vi "Bus Interface.vi"(0 "niUSRP Rx Core v1 FPGA":refnum<class "niUSRP Sync v1 FPGA.lvclass">, 1 "abort":bool, 5 "instruction":T2, 9 "input valid":bool) -> (6 "response":T1, 10 "done":bool, 14 "ready for input":bool)   [LabVIEW 2025, in "niUSRP Sync v1 FPGA.lvclass"]
uses:
  niUSRP Sync v1 FPGA.lvclass
  <instrlib>/_niInstr/Instruction Framework/v1/FPGA/Interfaces/Address Space/Address Space Instruction.ctl
  <instrlib>/_niInstr/Instruction Framework/v1/FPGA/Typedefs/Response.ctl
  niUSRP Sync v1 FPGA.lvclass/niUSRP Sync v1 FPGA.ctl
  <vilib>/rvi/DataTransferAndStorage/Container/Common/niFpgaContainerExecOnDevCompGetState.vi
  <vilib>/rvi/Emulation/niFpgaEmulationIsFPGAContextNoSignature.vi
  <vilib>/rvi/DataTransferAndStorage/Container/Common/niFpgaContainerGetUniqueNameForEmu.vi
  <vilib>/rvi/Memory/Memory_Emulation/niFpgaMemoryEmulationCacheClearOnFirstRun.vi
  <vilib>/rvi/Memory/Memory_Emulation/nirvimemoryEmulationManagerCache_MakeExclusive.vi
  <vilib>/rvi/Memory/Memory_Emulation/niFpgaMemoryEmulationValidateCache.vi
  <vilib>/rvi/Memory/Memory_Emulation/nirvimemoryEmulationManagerCache_InsertValue.vi
  <vilib>/Utility/error.llb/Clear Errors.vi
  <vilib>/rvi/Memory/Memory_Emulation/nirvimemoryEmulationManagerCache_ReleaseExclusive.vi
  <vilib>/rvi/Memory/Memory_Emulation/nirvimemoryEmulationManagerCache_GetValue.vi
  <vilib>/rvi/Memory/Memory_Emulation/nirvimemoryEmulationManagerCache_SetValue.vi
  <vilib>/rvi/Emulation/niFpgaProcessEmulError.vi
  <vilib>/rvi/Emulation/niFpgaSctlEmulationGetInTimedLoop.vi
  <vilib>/rvi/DataTransferAndStorage/Container/XNode/niFpgaContainer.xnode
  <vilib>/rvi/DataTransferAndStorage/Register/Emulation/niFpgaRegisterEmulationRefIn.vi
  <instrlib>/_niInstr/Instruction Framework/v1/FPGA/Typedefs/niInstr Instruction Framework v1 FPGA.lvlib
  <instrlib>/_niInstr/Basic Elements/v1/FPGA/niInstr Basic Elements v1 FPGA.lvlib
  <instrlib>/_niInstr/Instruction Framework/v1/FPGA/Interfaces/Address Space/Address Space.lvclass
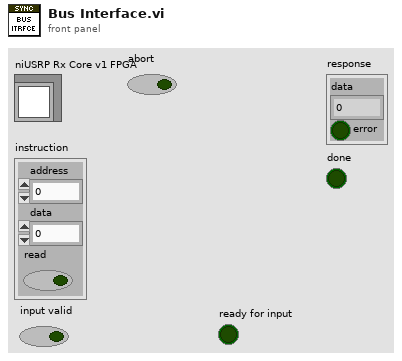
[diagram p1: front panel]
types:
  T1 = typedef "niInstr Instruction Framework v1 FPGA.lvlib/Response.ctl" = cluster{"data":u64, "error":bool}
  T2 = typedef "niInstr Instruction Framework Interfaces v1 FPGA.lvlib/Address Space.lvclass/Address Space Instruction.ctl" = cluster{"address":u32, "data":u64, "read":bool}
  T3 = typedef "niUSRP Sync v1 FPGA.lvclass/Regs.ctl" = cluster{"reset":refnum<k21>, "trigger enable":refnum<k21>, "trigger sync enable":refnum<k21>, "software trigger":refnum<k21>, "trigger select (U8)":refnum<k21>, "trigger out latch 0":refnum<k21>, "trigger out latch 1":refnum<k21>, "trigger time":refnum<k21>, "set trigger time":refnum<k21>, "clear trigger time":refnum<k21>, "time trigger ready":refnum<k21>, "time trigger set in past":refnum<k21>}
  T4 = enum8{"Software", "Digital Edge", "Rx Start Trigger", "Tx Start Trigger", "Immediate", "Future Time Event"}
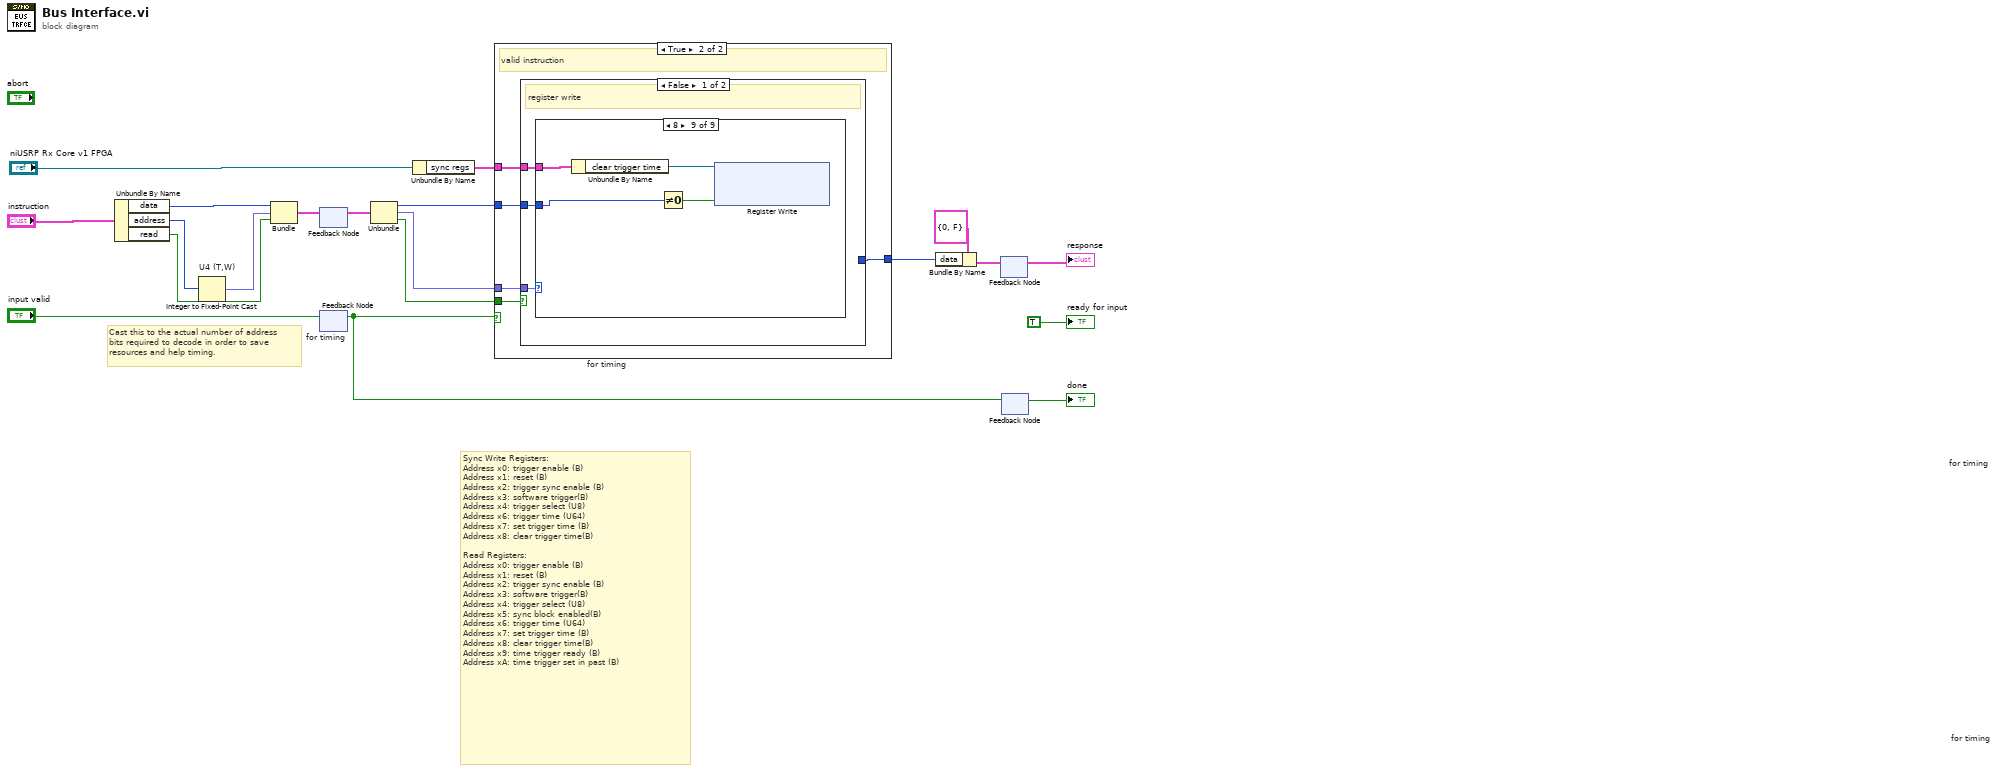
[diagram p0: block diagram]
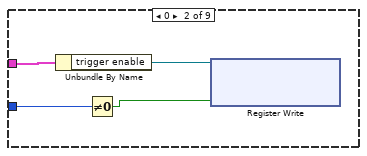
[diagram p4: hidden frame]
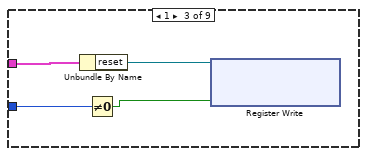
[diagram p5: hidden frame]
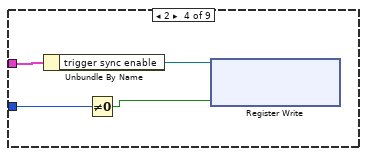
[diagram p6: hidden frame]
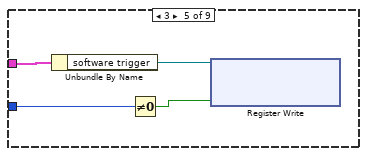
[diagram p7: hidden frame]
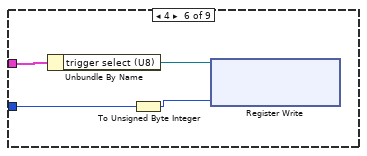
[diagram p8: hidden frame]
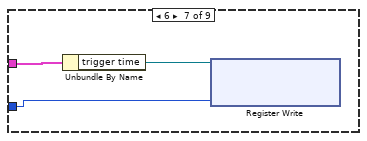
[diagram p9: hidden frame]
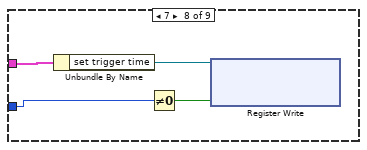
[diagram p10: hidden frame]
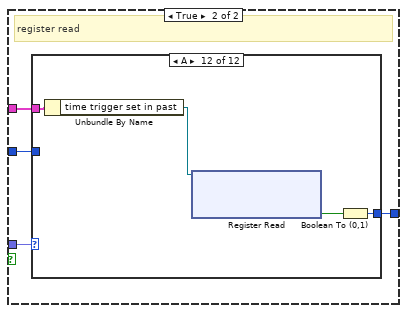
[diagram p11: hidden frame]
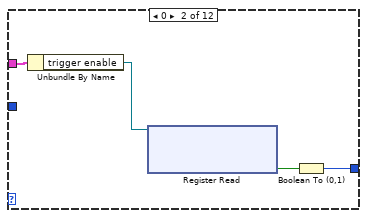
[diagram p13: hidden frame]
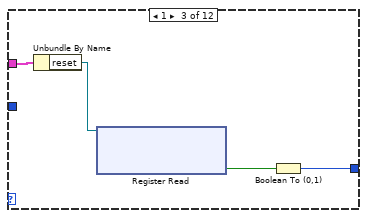
[diagram p14: hidden frame]
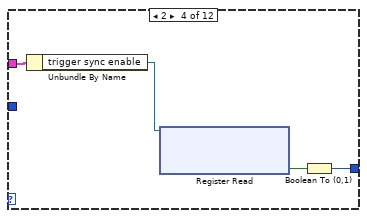
[diagram p15: hidden frame]
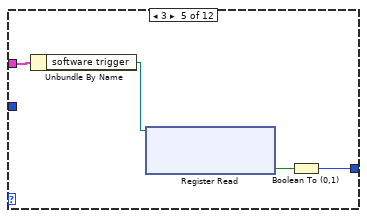
[diagram p16: hidden frame]
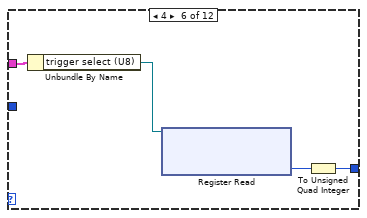
[diagram p17: hidden frame]
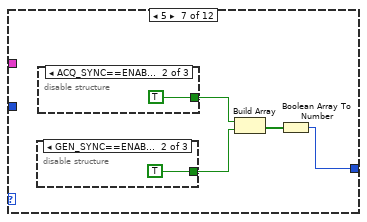
[diagram p18: hidden frame]
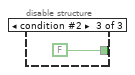
[diagram p20: hidden frame]
diagram:
  # "Sync Write Registers:\nAddress x0: trigger enable (B)\nAddress x1: reset (B)\nAddress x2: trigger sync enable (B)\nAddress x3: software trigger(B)\nAddress x4: trigger select (U8)\nAddress x6: trigger time (U64)\nAddress x7: set trigger time (B)\nAddress x8: clear trigger time(B)\n\nRead Registers:\nAddress x0: trigger enable (B)\nAddress x1: reset (B)\nAddress x2: trigger sync enable (B)\nAddress x3: software trigger(B)\nAddress x4: trigger select (U8)\nAddress x5: sync block enabled(B)\nAddress x6: trigger time (U64)\nAddress x7: set trigger time (B)\nAddress x8: clear trigger time(B)\nAddress x9: time trigger ready (B)\nAddress xA: time trigger set in past (B)"
  # "Cast this to the actual number of address\nbits required to decode in order to save\nresources and help timing."
  n1 = Unbundle By Name("instruction") -> ("data"=w17:u64, "address"=w20:u32, "read"=w15:bool)
  n2 = Integer to Fixed-Point Cast "U4 (T,W)"(integer=w20) -> (fixed-point=w16:fxp<+,4,4>)  [unwired: 1 in]
  n3 = Bundle("data"=w17, w16, "read"=w15) -> (w19:cluster{"data":u64, fxp<+,4,4>, "read":bool})  [unwired: 1 in]
  n4 = feedback #1 "for timing"() -> (w18:cluster{"data":u64, fxp<+,4,4>, "read":bool})  [unwired: 1 in]
  n5 = feedback-in #1(w19) -> ()
  n6 = feedback #2 "for timing"() -> (w1:bool)  [unwired: 1 in]
  n7 = feedback-in #2("input valid") -> ()
  n8 = Unbundle(w18) -> ("data"=w8:u64, w9:fxp<+,4,4>, "read"=w10:bool)
  n9 = Unbundle By Name("niUSRP Rx Core v1 FPGA") -> ("sync regs"=w11:T3)
  n10 = case shown="True" w1 {
    tunnel: w11 -> [_ w25]
    tunnel: w10 -> [_ w24]
    tunnel: w9 -> [_ w23]
    tunnel: w8 -> [_ w22]
    tunnel: [_ w21] -> w7
    frame False {
      # "invalid instruction"
    }
    frame True {
      # "valid instruction"
      n11 = case shown="False" w24 {
        tunnel: w23 -> [w28 w63]
        tunnel: [_ w60] -> w21
        tunnel: w22 -> [w27 w62]
        tunnel: w25 -> [w26 w61]
        frame False {
          # "register write"
          n12 = case shown="8" w28 {
            tunnel: w27 -> [_ w30 w34 w38 w42 w46 w49 w53 w57]
            tunnel: w26 -> [_ w31 w35 w39 w43 w47 w50 w54 w58]
            frame Default {
              # "non-existent register"
            }
            frame 0 {
              n13 = Unbundle By Name(w31) -> ("trigger enable"=w32:refnum<k21>)
              n14 = Not Equal To 0?(x=w30) -> (x != 0?=w29:bool)
              n15 = xnode ("Register Write")("Data"=w29, "Register In"=w32) -> ()  [unwired: 1 out]
            }
            frame 1 {
              n16 = Unbundle By Name(w35) -> ("reset"=w36:refnum<k21>)
              n17 = Not Equal To 0?(x=w34) -> (x != 0?=w33:bool)
              n18 = xnode ("Register Write")("Data"=w33, "Register In"=w36) -> ()  [unwired: 1 out]
            }
            frame 2 {
              n19 = Unbundle By Name(w39) -> ("trigger sync enable"=w40:refnum<k21>)
              n20 = Not Equal To 0?(x=w38) -> (x != 0?=w37:bool)
              n21 = xnode ("Register Write")("Data"=w37, "Register In"=w40) -> ()  [unwired: 1 out]
            }
            frame 3 {
              n22 = Unbundle By Name(w43) -> ("software trigger"=w44:refnum<k21>)
              n23 = Not Equal To 0?(x=w42) -> (x != 0?=w41:bool)
              n24 = xnode ("Register Write")("Data"=w41, "Register In"=w44) -> ()  [unwired: 1 out]
            }
            frame 4 {
              n25 = Unbundle By Name(w47) -> ("trigger select (U8)"=w48:refnum<k21>)
              n26 = To Unsigned Byte Integer(number=w46) -> (unsigned 8bit integer=w45:u8)
              n27 = xnode ("Register Write")("Data"=w45, "Register In"=w48) -> ()  [unwired: 1 out]
            }
            frame 6 {
              n28 = Unbundle By Name(w50) -> ("trigger time"=w51:refnum<k21>)
              n29 = xnode ("Register Write")("Data"=w49, "Register In"=w51) -> ()  [unwired: 1 out]
            }
            frame 7 {
              n30 = Unbundle By Name(w54) -> ("set trigger time"=w55:refnum<k21>)
              n31 = Not Equal To 0?(x=w53) -> (x != 0?=w52:bool)
              n32 = xnode ("Register Write")("Data"=w52, "Register In"=w55) -> ()  [unwired: 1 out]
            }
            frame 8 {
              n33 = Unbundle By Name(w58) -> ("clear trigger time"=w59:refnum<k21>)
              n34 = Not Equal To 0?(x=w57) -> (x != 0?=w56:bool)
              n35 = xnode ("Register Write")("Data"=w56, "Register In"=w59) -> ()  [unwired: 1 out]
            }
          }
        }
        frame True {
          # "register read"
          n36 = case shown="A" w63 {
            tunnel: w62 -> [_ _ _ _ _ _ _ _ _ _ _ _]
            tunnel: w61 -> [_ w66 w70 w74 w79 w82 _ w96 w100 w104 w108 w112]
            tunnel: [_ w64 w68 w72 w78 w80 w84 w97 w99 w103 w107 w111] -> w60
            frame Default {
              # "non-existent register"
            }
            frame 0 {
              n37 = Unbundle By Name(w66) -> ("trigger enable"=w67:refnum<k21>)
              n38 = xnode ("Register Read")("Register In"=w67) -> ("Data"=w65:bool)  [unwired: 1 out]
              n39 = Boolean To (0,1)(Boolean=w65) -> (0, 1=w64:i16)
            }
            frame 1 {
              n40 = Unbundle By Name(w70) -> ("reset"=w71:refnum<k21>)
              n41 = xnode ("Register Read")("Register In"=w71) -> ("Data"=w69:bool)  [unwired: 1 out]
              n42 = Boolean To (0,1)(Boolean=w69) -> (0, 1=w68:i16)
            }
            frame 2 {
              n43 = Unbundle By Name(w74) -> ("trigger sync enable"=w75:refnum<k21>)
              n44 = xnode ("Register Read")("Register In"=w75) -> ("Data"=w73:bool)  [unwired: 1 out]
              n45 = Boolean To (0,1)(Boolean=w73) -> (0, 1=w72:i16)
            }
            frame 3 {
              n46 = Unbundle By Name(w79) -> ("software trigger"=w77:refnum<k21>)
              n47 = xnode ("Register Read")("Register In"=w77) -> ("Data"=w76:bool)  [unwired: 1 out]
              n48 = Boolean To (0,1)(Boolean=w76) -> (0, 1=w78:i16)
            }
            frame 4 {
              n49 = Unbundle By Name(w82) -> ("trigger select (U8)"=w83:refnum<k21>)
              n50 = xnode ("Register Read")("Register In"=w83) -> ("Data"=w81:T4)  [unwired: 1 out]
              n51 = To Unsigned Quad Integer(1:w81) -> (0:w80:u64)
            }
            frame 5 {
              n52 = disable-structure shown="GEN_SYNC==ENABLED" {
                disable-tunnel: [_ TRUE FALSE] -> w85
                frame condition #0 {
                  w89 = TRUE ("assert")
                  w88 = -1074101118  # BasicElementsCodegenError
                  # "IF YOU UNEXPECTEDLY REACH THIS STATE:\nlabview has failed to propagate the conditional symbol for this structure. to fix this, edit the condition and click OK (typically, no actual changes are necessary)."
                  n53 = call <instrlib>:"Assert.vi"("assert"=w89, "error code"=w88, "enable show error"=w89) -> ()  [unwired: 13 in]
                }
                frame condition #1 (active) {
                }
                frame condition #2 {
                }
              }
              n54 = disable-structure shown="ACQ_SYNC==ENABLED" {
                disable-tunnel: [_ TRUE FALSE] -> w86
                frame condition #0 {
                  w93 = TRUE ("assert")
                  w92 = -1074101118  # BasicElementsCodegenError
                  # "IF YOU UNEXPECTEDLY REACH THIS STATE:\nlabview has failed to propagate the conditional symbol for this structure. to fix this, edit the condition and click OK (typically, no actual changes are necessary)."
                  n55 = call <instrlib>:"Assert.vi"("assert"=w93, "error code"=w92, "enable show error"=w93) -> ()  [unwired: 13 in]
                }
                frame condition #1 (active) {
                }
                frame condition #2 {
                }
              }
              n56 = Build Array(w86, w85) -> (w87:bool[])
              n57 = Boolean Array To Number(Boolean array=w87) -> (number=w84:u32)
            }
            frame 6 {
              n58 = Unbundle By Name(w96) -> ("trigger time"=w98:refnum<k21>)
              n59 = xnode ("Register Read")("Register In"=w98) -> ("Data"=w97:u64)  [unwired: 1 out]
            }
            frame 7 {
              n60 = Unbundle By Name(w100) -> ("set trigger time"=w102:refnum<k21>)
              n61 = xnode ("Register Read")("Register In"=w102) -> ("Data"=w101:bool)  [unwired: 1 out]
              n62 = Boolean To (0,1)(Boolean=w101) -> (0, 1=w99:i16)
            }
            frame 8 {
              n63 = Unbundle By Name(w104) -> ("clear trigger time"=w106:refnum<k21>)
              n64 = xnode ("Register Read")("Register In"=w106) -> ("Data"=w105:bool)  [unwired: 1 out]
              n65 = Boolean To (0,1)(Boolean=w105) -> (0, 1=w103:i16)
            }
            frame 9 {
              n66 = Unbundle By Name(w108) -> ("time trigger ready"=w110:refnum<k21>)
              n67 = xnode ("Register Read")("Register In"=w110) -> ("Data"=w109:bool)  [unwired: 1 out]
              n68 = Boolean To (0,1)(Boolean=w109) -> (0, 1=w107:i16)
            }
            frame 10 {
              n69 = Unbundle By Name(w112) -> ("time trigger set in past"=w114:refnum<k21>)
              n70 = xnode ("Register Read")("Register In"=w114) -> ("Data"=w113:bool)  [unwired: 1 out]
              n71 = Boolean To (0,1)(Boolean=w113) -> (0, 1=w111:i16)
            }
          }
        }
      }
    }
  }
  n72 = Bundle By Name(cluster=T1 {"data"=0, "error"=FALSE} ("response"), "data"=w7) -> (w4:T1)
  n73 = feedback #3 "for timing"() -> (→"response":T1)  [unwired: 1 in]
  n74 = feedback-in #3(w4) -> ()
  n75 = feedback #4 "for timing"() -> (→"done":bool)  [unwired: 1 in]
  n76 = feedback-in #4(w1) -> ()
  "ready for input" <- TRUE ("ready for input")
